vi "Handle Command.vi"(8 "error in (no error)":errorcluster, 9 "Value":bool, 11 "Valve in":refnum<class "ValueSetControl.lvclass">) -> (0 "error out":errorcluster, 3 "Valve out":refnum<class "ValueSetControl.lvclass">)   [LabVIEW 2023, in "VolatusControl.lvlib" / "ValueSetControl.lvclass"]
uses:
  ValueSetControl.lvclass
  ValueSetControl.lvclass/ValueSetControl.ctl
  messages/CmdAnalog/Data.ctl
  Volatus/MessageQ/MessageQ.lvclass/MessageQ.ctl
  Volatus/MessageQ/MessageQ.lvclass
  messages/CmdAnalog/CmdAnalog.lvlib
  messages/CmdAnalogMultiple/CmdAnalogMultiple.lvlib
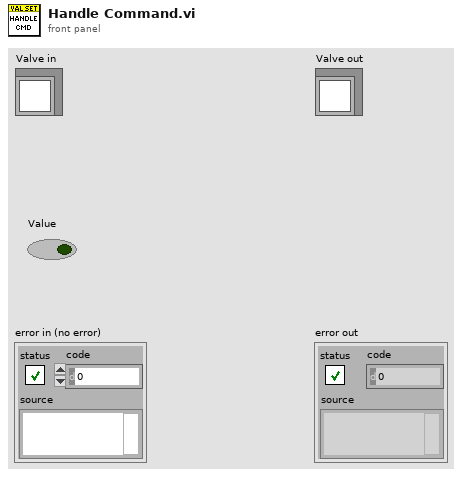
[diagram p1: front panel]
types:
  T1 = typedef "CmdAnalog.lvlib/Data.ctl" = cluster{"channel":string, "value":dbl}
  T2 = typedef "CmdAnalogMultiple.lvlib/Data.ctl" = cluster{"values":T1[]}
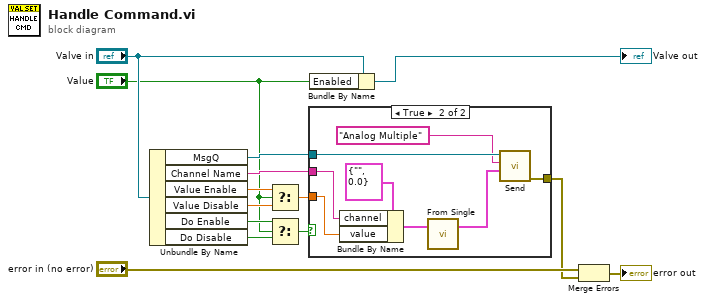
[diagram p0: block diagram]
diagram:
  n1 = Unbundle By Name("Valve in") -> ("MsgQ"=w5:refnum<class "MessageQ.lvclass">, "Channel Name"=w6:string, "Value Enable"=w12:dbl, "Value Disable"=w11:dbl, "Do Enable"=w10:bool, "Do Disable"=w9:bool)
  n2 = Select(t=w12, s="Value", f=w11) -> (s? t:f=w7:dbl)
  n3 = Select(t=w10, s="Value", f=w9) -> (s? t:f=w8:bool)
  n4 = case shown="True" w8 {
    tunnel: w7 -> [_ w19]
    tunnel: w6 -> [_ w20]
    tunnel: w5 -> [_ w22]
    tunnel: [_ w16] -> w3
    frame False {
    }
    frame True {
      n5 = Bundle By Name(cluster=T1 {"channel"="", "value"=0.0} ("CmdAnalog"), "channel"=w20, "value"=w19) -> (w18:T1)
      n6 = call "From Single.vi"("CmdAnalog"=w18) -> ("CmdAnalogMultiple"=w15:T2)  [unwired: 6 in]
      n7 = call "Send.vi"("Data"=w15, "ID"="Analog Multiple", "MessageQ in"=w22) -> ("error out"=w16:errorcluster)  [unwired: 7 in, 1 out]
    }
  }
  n8 = Bundle By Name(cluster="Valve in", "Enabled"="Value") -> (→"Valve out":refnum<class "ValueSetControl.lvclass">)
  n9 = Merge Errors("error in (no error)", w3) -> (→"error out":errorcluster)
